vi "Write Channels_ Reference.vi"(8 "error in (no error)":errorcluster, 10 "Channels: Lockin":T1={"Ch"=[1], " f (Hz)"=[13.0], "Phase (°)"=[0.0], "TC (s)"=[0.1], "order"=[2]} {"TC (s)" format="%#_3p"; "Phase (°)" format="%#_3g"}, 11 "LockinDAQ":refnum<class "LockinDAQ.lvclass">) -> (0 "error out":errorcluster, 3 "LockinDAQ out":refnum<class "LockinDAQ.lvclass">)   [LabVIEW 2016, in "LockinDAQ.lvclass"]
uses:
  LockinDAQ.lvclass
  Typedefs/REF-cluster.ctl
  LockinDAQ.lvclass/LockinDAQ.ctl
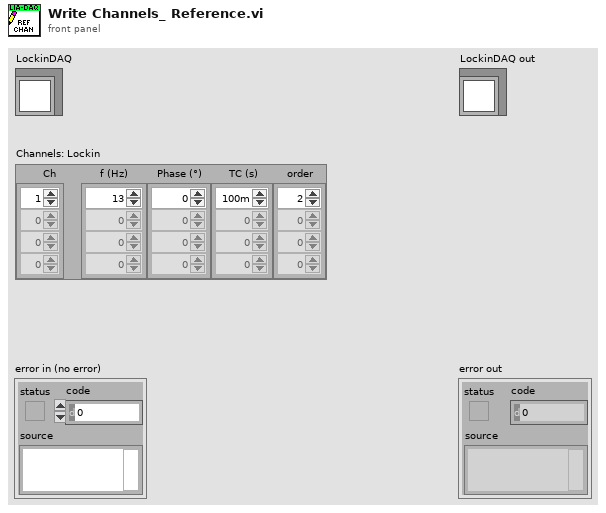
[diagram p1: front panel]
types:
  T1 = typedef "LockinDAQ.lvclass/REF-cluster.ctl" = cluster{"Ch":i32[], " f (Hz)":dbl[], "Phase (°)":dbl[], "TC (s)":dbl[], "order":i32[]}
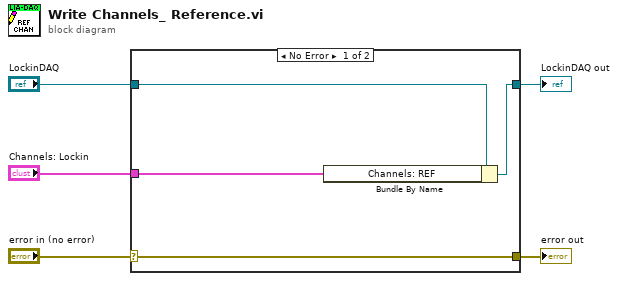
[diagram p0: block diagram]
diagram:
  n1 = case shown="No Error" "error in (no error)" {
    selector: "error in (no error)" -> [w9 w10]
    tunnel: [w9 w10] -> w4
    tunnel: [w7 w11] -> w2
    tunnel: "LockinDAQ" -> [w8 w11]
    tunnel: "Channels: Lockin" -> [w6 _]
    frame No Error {
      n2 = Bundle By Name(cluster=w8, "Channels: REF"=w6) -> (w7:refnum<class "LockinDAQ.lvclass">)
    }
    frame Error {
    }
  }
  "error out" <- w4
  "LockinDAQ out" <- w2
